vi "Pre-Build Action.vi"(6 "Top Level/Always Included VIs":path[](array[path]), 7 "Main Destination Path":path, 9 "Target Name":string, 10 "Build Specification Name":string, 11 "Project Path":path) -> (0 "error out":errorcluster)   [LabVIEW 2014]
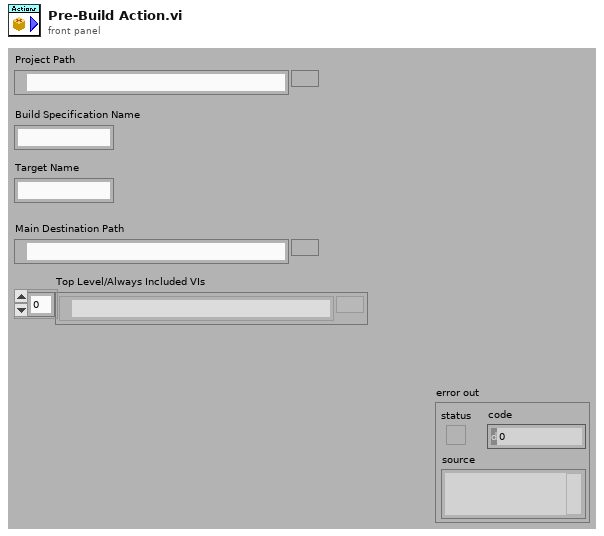
[diagram p1: front panel]
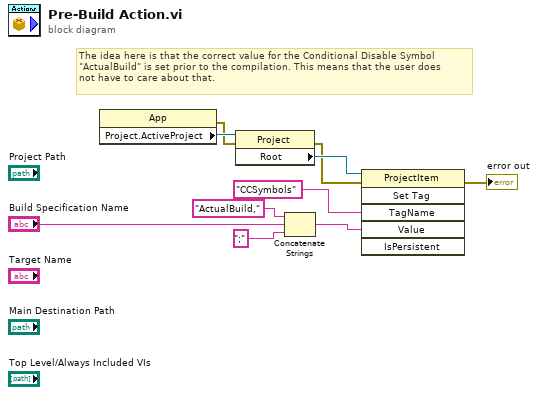
[diagram p0: block diagram]
diagram:
  # "The idea here is that the correct value for the Conditional Disable Symbol\n\"ActualBuild\" is set prior to the compilation. This means that the user does\nnot have to care about that."
  n1 = property class="App"() -> (error out=w3:errorcluster, "Project.ActiveProject"=w10:refnum<vi>)  [unwired: 2 in, 1 out]
  n2 = property class="Project"(reference=w10, error in=w3) -> (error out=w2:errorcluster, "Root"=w9:refnum<vi>)  [unwired: 1 out]
  n3 = Concatenate Strings("ActualBuild," ("Tag Name"), "Build Specification Name", ";" ("string")) -> (w6:string)
  n4 = invoke class="ProjectItem" method="Set Tag"(reference=w9, error in=w2, "TagName"="CCSymbols" ("Tag Name"), "Value"=w6) -> (error out=→"error out":errorcluster)  [unwired: 2 in, 5 out]
